vi "test_ConflictingNameInProject_CheckPluginNameIsValid_NameInvalid.vi"() -> (6 "pass":bool, 8 "result":string, 15 "error out":errorcluster)   [LabVIEW 2021]
uses:
  <vilib>/ErrorRing/Error Ring.xnode
  Generator/_Editor/MeasurementService Editor.lvlib
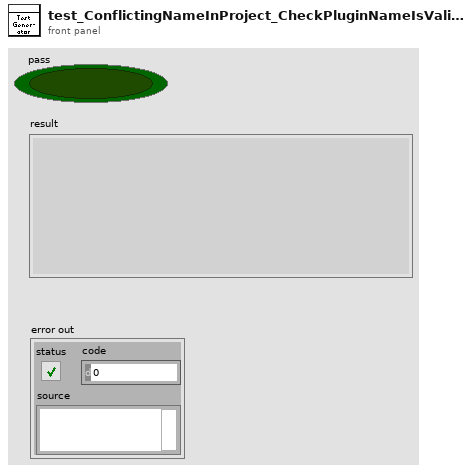
[diagram p1: front panel]
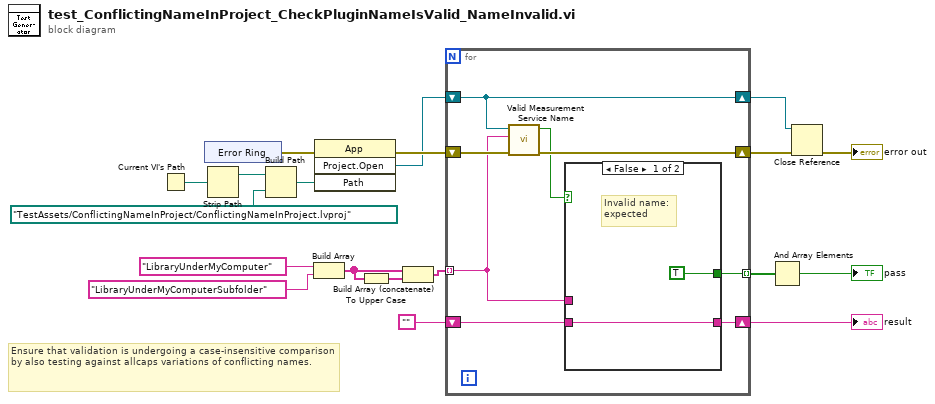
[diagram p0: block diagram]
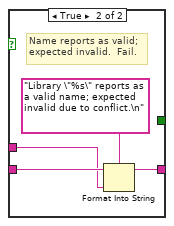
[diagram p2: hidden frame]
diagram:
  # "Ensure that validation is undergoing a case-insensitive comparison by also testing against allcaps variations of conflicting names."
  n1 = Current VI's Path() -> (path=w19:path)
  n2 = xnode "Error Ring"() -> ("error out"=w16:errorcluster)
  n3 = Strip Path(path=w19) -> (stripped path=w18:path)  [unwired: 1 out]
  n4 = Build Path(base path=w18, name or relative path=path "TestAssets/ConflictingNameInProject/ConflictingNameInProject.lvproj" ("path")) -> (appended path=w15:path)
  n5 = Build Array("LibraryUnderMyComputer", "LibraryUnderMyComputerSubfolder") -> (w1:string[])
  n6 = invoke class="App" method="Project.Open"(error in=w16, "Path"=w15) -> (error out=w7:errorcluster, "Project:Open"=w6:refnum<vi>)  [unwired: 2 in, 2 out]
  n7 = To Upper Case(1:w1) -> (0:w2:string[])
  n8 = Build Array (concatenate)(w1, w2) -> (w3:string[])
  n9 = for {
    shift-right: [w26] -> w14
    shift-left: w7 -> [w27]
    tunnel: w3 -> [w20] mode=indexing
    shift-right: [w25] -> w12
    shift-left: w6 -> [w25]
    shift-right: [w22] -> w10
    shift-left: "" -> [w23]
    tunnel: [w21] -> w9 mode=indexing
    n10 = call "Valid Measurement Service Name.vi"("error in"=w27, "requested plugin name"=w20, "project ref"=w25) -> ("error out"=w26:errorcluster, "valid name?"=w24:bool)  [unwired: 7 in]
    n11 = case shown="False" w24 {
      tunnel: w23 -> [w29 w33]
      tunnel: [w29 w32] -> w22
      tunnel: [TRUE _] -> w21
      tunnel: w20 -> [_ w31]
      frame False {
        # "Invalid name:\nexpected"
      }
      frame True {
        # "Name reports as valid;\nexpected invalid.  Fail."
        n12 = Format Into String(format string="Library \"%s\" reports as a valid name; expected invalid due to conflict.\n", initial string=w33, w31) -> (resulting string=w32:string)  [unwired: 1 in, 1 out]
      }
    }
  }
  "result" <- w10
  n13 = And Array Elements(Boolean array=w9) -> (logical AND=→"pass":bool)
  n14 = Close Reference(reference=w12, error in (no error)=w14) -> (error out=→"error out":errorcluster)
